vi "DAQ Assist Input 2.vi"() -> (7 "?":bool[](array[boolean]))   [LabVIEW 2015]
panel:
  out "error out":errorcluster
  in  "device name":tag="Dev2"
  in  "error in":errorcluster
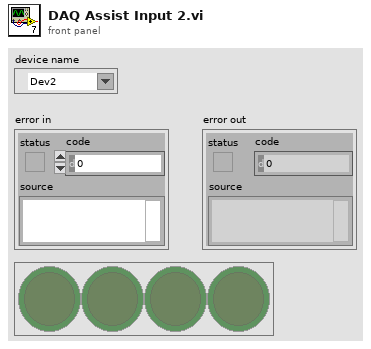
[diagram p1: front panel]
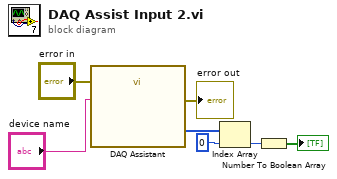
[diagram p0: block diagram]
diagram:
  n1 = call "DAQ Assistant"("error in"="error in", "device name"="device name") -> ("data"=w1:u32[], "error out"=→"error out":errorcluster)  [unwired: 15 in, 1 out]
  n2 = Index Array(array=w1, index=0) -> (element=w3:u32)
  n3 = Number To Boolean Array(number=w3) -> (Boolean array=→"?":bool[])
